vi "Send Return Self.vi"(7 "Message Priority (Normal)":T1=enum."Normal", 8 "error in (no error)":errorcluster, 9 "timeout in ms (5000)":i32=5000, 11 "Message Enqueuer":refnum<class "Message Enqueuer.lvclass">) -> (0 "error out":errorcluster, 2 "cRIO-CO2 class":refnum<class "cRIO-CO2.lvclass">, 3 "Message Enqueuer out":refnum<class "Message Enqueuer.lvclass">)   [LabVIEW 2015, in "cRIO-Carbondioxide.lvlib" / "cRIO-CO2.lvlib" / "Return Self.lvclass"]
doc: "This VI sends the message to an actor."
uses:
  Return Self.lvclass
  <vilib>/ActorFramework/Message Enqueuer/Message Enqueuer.lvclass
  <vilib>/ActorFramework/Message Enqueuer/Message Priority.ctl
  cRIO-CO2/cRIO-CO2.lvclass
  Return Self.lvclass/Return Self.ctl
  <vilib>/ActorFramework/Message Enqueuer/Message Enqueuer.lvclass/Message Enqueuer.ctl
  <vilib>/ActorFramework/Message Priority Queue/Priority Enqueue.vi
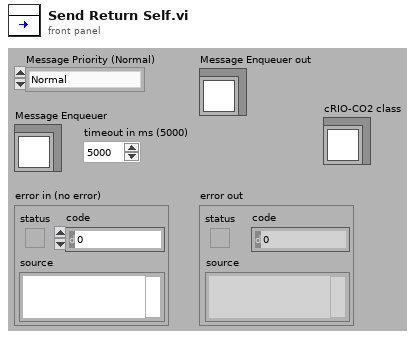
[diagram p1: front panel]
types:
  T1 = typedef "Actor Framework.lvlib/Message Enqueuer.lvclass/Message Priority.ctl" = enum16{"Low", "Normal", "High"}
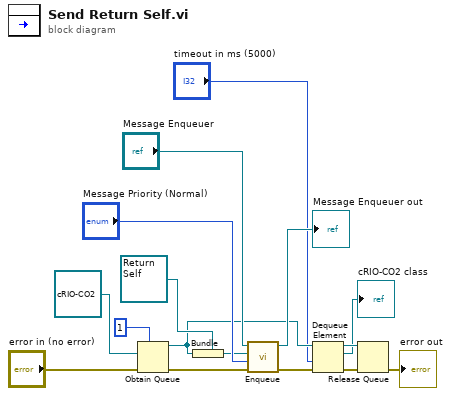
[diagram p0: block diagram]
diagram:
  n1 = Obtain Queue(max queue size (-1, unlimited)=1, element data type=refnum<class "cRIO-CO2.lvclass"> refnum ("cRIO-CO2.lvclass"), error in (no error)="error in (no error)") -> (queue out=w6:refnum<queue>, error out=w14:errorcluster)  [unwired: 2 in, 1 out]
  n2 = Bundle(cluster=refnum<class "Return Self.lvclass"> refnum ("Object"), w6) -> (w10:refnum<class "Return Self.lvclass">)
  n3 = call <vilib>:"Enqueue.vi"("error in (no error)"=w14, "Message Priority (Normal)"="Message Priority (Normal)", "Message"=w10, "Message Enqueuer in"="Message Enqueuer") -> ("error out"=w7:errorcluster, "Message Enqueuer out"=→"Message Enqueuer out":refnum<class "Message Enqueuer.lvclass">)  [unwired: 6 in]
  n4 = Dequeue Element(queue=w6, timeout in ms (-1)="timeout in ms (5000)", error in (no error)=w7) -> (queue out=w2:refnum<queue>, element=→"cRIO-CO2 class":refnum<class "cRIO-CO2.lvclass">, error out=w4:errorcluster)  [unwired: 1 out]
  n5 = Release Queue(queue=w2, error in (no error)=w4) -> (error out=→"error out":errorcluster)  [unwired: 1 in, 2 out]
